vi "Set Waveform to Constant.vi"(8 "Error In":errorcluster, 9 "Original Waveform":waveform(dbl), 10 "New Value":dbl) -> (0 "Error Out":errorcluster, 1 "New Waveform":waveform(dbl))   [LabVIEW 2020]
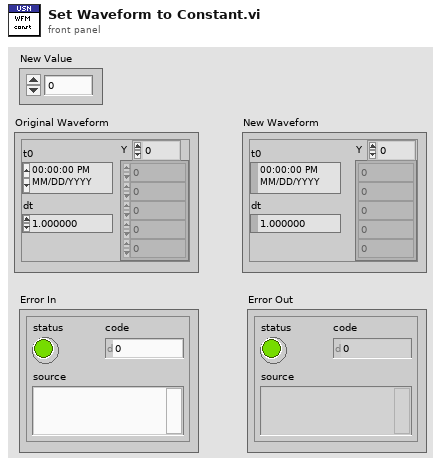
[diagram p1: front panel]
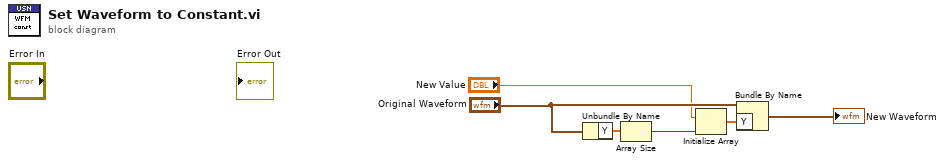
[diagram p0: block diagram]
diagram:
  n1 = Unbundle By Name("Original Waveform") -> ("Y"=w4:dbl[])
  n2 = Array Size(array=w4) -> (size(s)=w5:i32)
  n3 = Initialize Array("New Value", w5) -> (w6:dbl[])
  n4 = Bundle By Name(cluster="Original Waveform", "Y"=w6) -> (→"New Waveform":waveform(dbl))
